vi "Gerilim_Tablo_Doldur.vi"(10 "Table Reference in":refnum<vi>, 11 "appended array in":dbl[][](array[numeric])=[[0.12345, 1.2, 0.12345], [0.12345, 1.2, 0.12345], [0.12345, 0.12345, 0.12345], [0.12345, 0.12345, 0.12345]]) -> (1 "Test Result":bool=TRUE, 2 "Table Values":string[][](array[string])=[["0,123", "0,1235"], ["0,123", "0,1235"], ["0,123", "0,1235"], ["0,123", "0,1235"], ["0,050", "0,0000"]], 3 "appended array Out":dbl[][](array[numeric])=[[0.12345, 1.2, 0.12345], [0.12345, 1.2, 0.12345], [0.12345, 0.12345, 0.12345], [0.12345, 0.12345, 0.12345], [0.049999999999999996, 0.0, 0.0]])   [LabVIEW 2014]
uses:
  TestStandInteraction/VeriPaylasim_Globali.vi
panel:
  out "OlcumNo":u16=6
  out "appended array":dbl[](array[numeric])=[0.049999999999999996, 0.0, 0.0, 0.0, 0.0, 0.0, 0.0, 0.05]
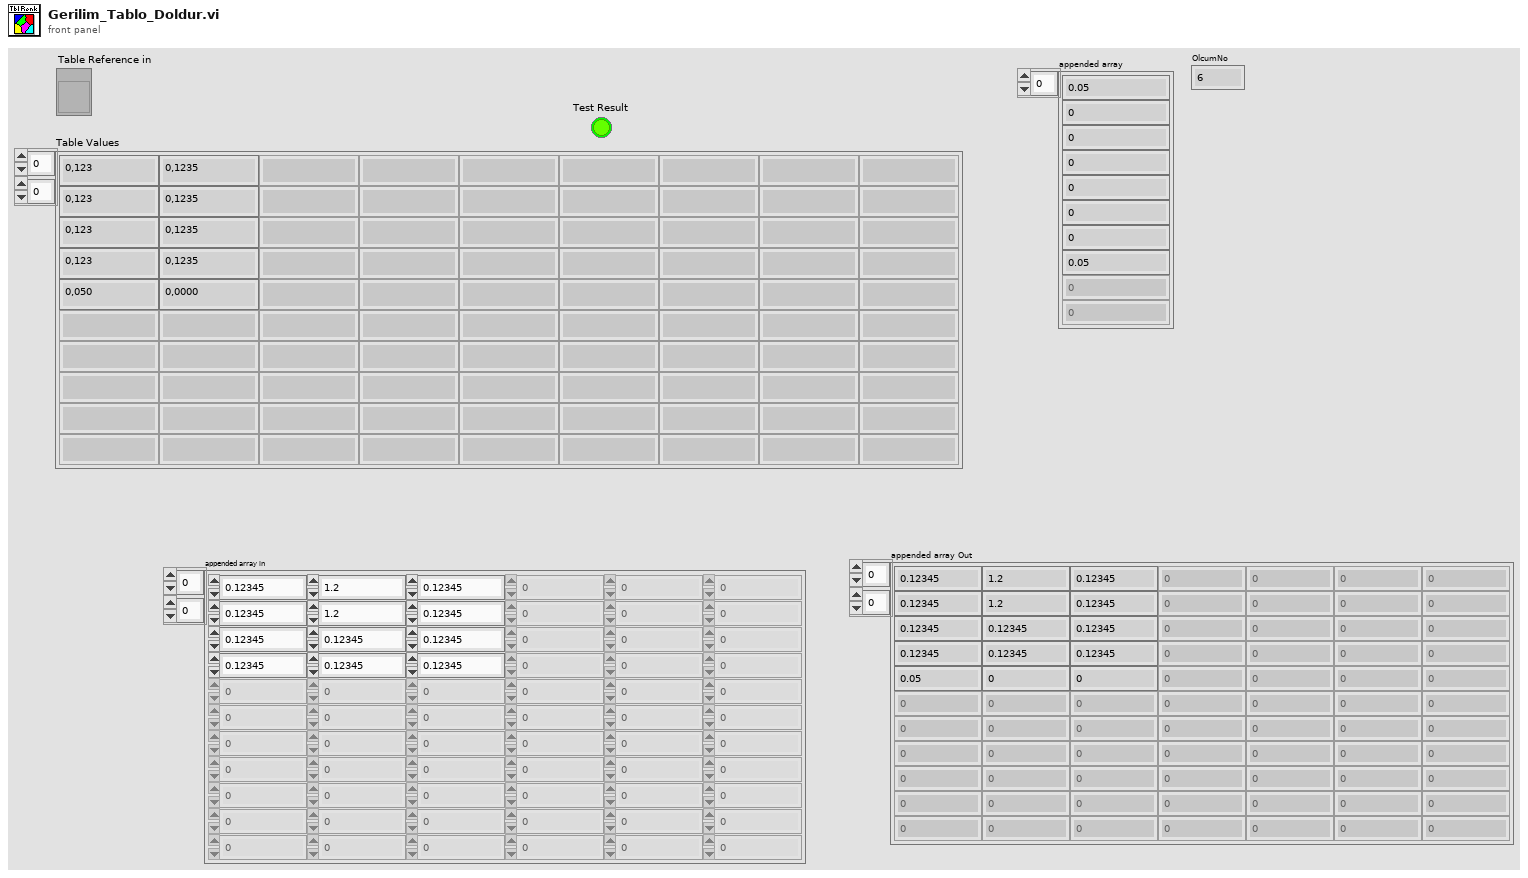
[diagram p1: front panel]
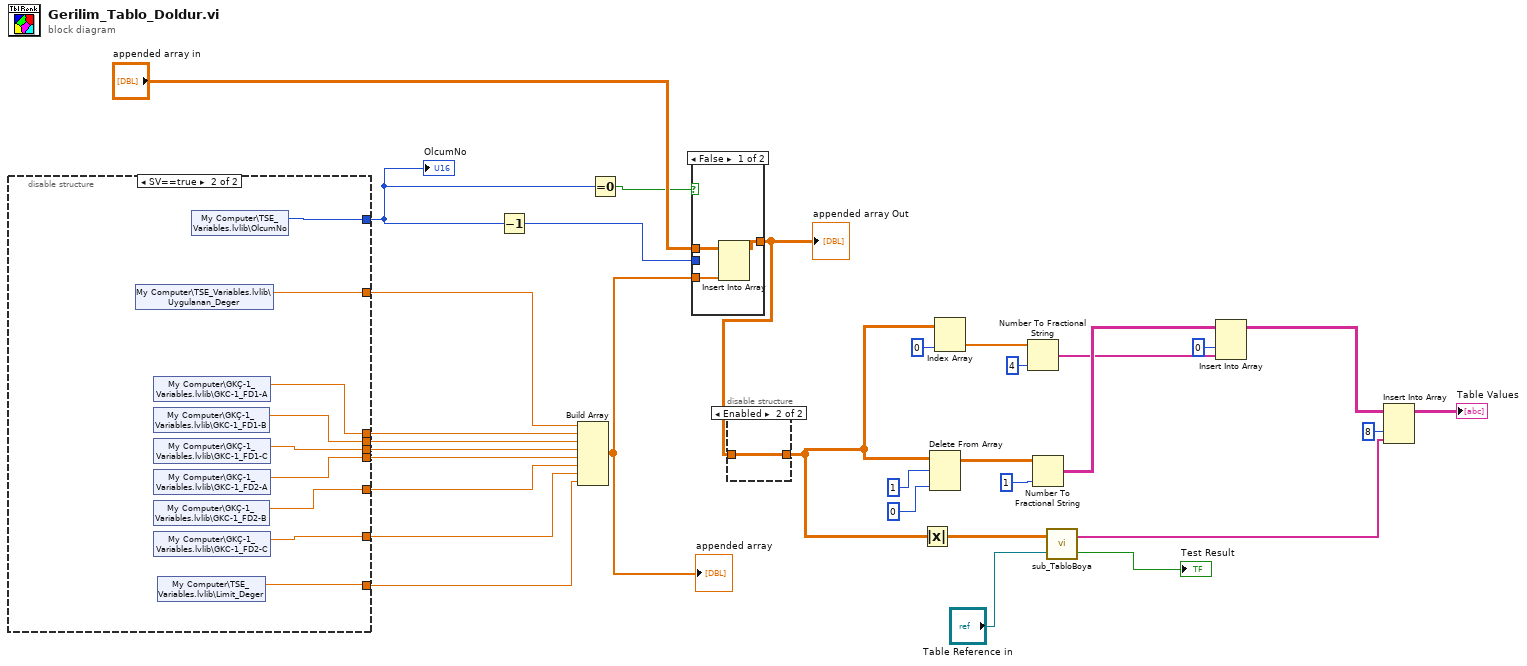
[diagram p0: block diagram]
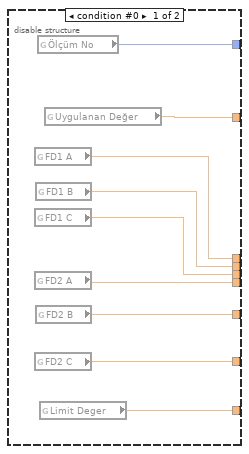
[diagram p2: hidden frame]
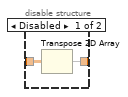
[diagram p4: hidden frame]
diagram:
  n1 = disable-structure shown="SV==true" {
    disable-tunnel: [w41 w50] -> w21
    disable-tunnel: [w40 w49] -> w20
    disable-tunnel: [w39 w47] -> w8
    disable-tunnel: [w38 w46] -> w7
    disable-tunnel: [w37 w48] -> w6
    disable-tunnel: [w36 w42] -> w5
    disable-tunnel: [w35 w43] -> w4
    disable-tunnel: [w34 w44] -> w3
    disable-tunnel: [w33 w45] -> w2
    frame condition #0 {
      n2 = global read "VeriPaylasim_Globali.vi" "FD1 A"() -> (w39:dbl)
      n3 = global read "VeriPaylasim_Globali.vi" "FD1 C"() -> (w33:dbl)
      n4 = global read "VeriPaylasim_Globali.vi" "FD2 A"() -> (w34:dbl)
      n5 = global read "VeriPaylasim_Globali.vi" "FD2 C"() -> (w36:dbl)
      n6 = global read "VeriPaylasim_Globali.vi" "FD1 B"() -> (w38:dbl)
      n7 = global read "VeriPaylasim_Globali.vi" "FD2 B"() -> (w35:dbl)
      n8 = global read "VeriPaylasim_Globali.vi" "Ölçüm No"() -> (w41:u16)
      n9 = global read "VeriPaylasim_Globali.vi" "Limit Deger"() -> (w37:dbl)
      n10 = global read "VeriPaylasim_Globali.vi" "Uygulanan Değer"() -> (w40:dbl)
    }
    frame condition #1 (active) {
      n11 = shared-variable "My Computer\\TSE_Variables.lvlib\\Uygulanan_Deger"() -> (w49:dbl)  [unwired: 1 in, 1 out]
      n12 = shared-variable "My Computer\\GKÇ-1_Variables.lvlib\\GKC-1_FD1-A"() -> (w47:dbl)  [unwired: 1 in, 1 out]
      n13 = shared-variable "My Computer\\GKÇ-1_Variables.lvlib\\GKC-1_FD1-B"() -> (w46:dbl)  [unwired: 1 in, 1 out]
      n14 = shared-variable "My Computer\\GKÇ-1_Variables.lvlib\\GKC-1_FD1-C"() -> (w45:dbl)  [unwired: 1 in, 1 out]
      n15 = shared-variable "My Computer\\GKÇ-1_Variables.lvlib\\GKC-1_FD2-A"() -> (w44:dbl)  [unwired: 1 in, 1 out]
      n16 = shared-variable "My Computer\\GKÇ-1_Variables.lvlib\\GKC-1_FD2-B"() -> (w43:dbl)  [unwired: 1 in, 1 out]
      n17 = shared-variable "My Computer\\GKÇ-1_Variables.lvlib\\GKC-1_FD2-C"() -> (w42:dbl)  [unwired: 1 in, 1 out]
      n18 = shared-variable "My Computer\\TSE_Variables.lvlib\\Limit_Deger"() -> (w48:dbl)  [unwired: 1 in, 1 out]
      n19 = shared-variable "My Computer\\TSE_Variables.lvlib\\OlcumNo"() -> (w50:u16)  [unwired: 1 in, 1 out]
    }
  }
  "OlcumNo" <- w21
  n20 = Decrement(x=w21) -> (x-1=w23:u16)
  n21 = Build Array(w20, w8, w7, w2, w3, w4, w5, w6) -> (w26:dbl[])
  "appended array" <- w26
  n22 = Equal To 0?(x=w21) -> (x = 0?=w22:bool)
  n23 = case shown="False" w22 {
    tunnel: w26 -> [w51 _]
    tunnel: [w52 w54] -> w25
    tunnel: "appended array in" -> [w53 w54]
    tunnel: w23 -> [_ _]
    frame False {
      n24 = Insert Into Array(array=w53, new element=w51) -> (w52:dbl[][])  [unwired: 2 in]
    }
    frame True {
    }
  }
  "appended array Out" <- w25
  n25 = disable-structure shown="Enabled" {
    disable-tunnel: [w56 w57] -> w17
    disable-tunnel: w25 -> [w55 w57]
    frame Disabled {
      n26 = Transpose 2D Array(2D array=w55) -> (transposed array=w56:dbl[][])
    }
    frame Enabled {
    }
  }
  n27 = Absolute Value(x=w17) -> (abs(x)=w1:dbl[][])
  n28 = Delete From Array "Delete From Array"(array=w17, length=1, index (col)=0 ("disabled index (col)")) -> (array with subset deleted=w14:dbl[][])  [unwired: 1 in, 1 out]
  n29 = Index Array "Index Array"(array=w17, index (col)=0 ("disabled index (col)")) -> (element=w18:dbl[])  [unwired: 1 in]
  n30 = Number To Fractional String(number=w18, precision (6)=i16 4) -> (F-format string=w11:string[])  [unwired: 2 in]
  n31 = Number To Fractional String(number=w14, precision (6)=i16 1) -> (F-format string=w12:string[][])  [unwired: 2 in]
  n32 = call "sub_TabloBoya.vi"("Table in"="Table Reference in", "Tablo Degerleri"=w1) -> ("Test Result"=→"Test Result":bool, "RESULTS"=w30:string[])
  n33 = Insert Into Array(array=w12, index (col)=0 ("disabled index (col)"), new element=w11) -> (w13:string[][])  [unwired: 1 in]
  n34 = Insert Into Array(array=w13, index (col)=8 ("disabled index (col)"), new element=w30) -> (→"Table Values":string[][])  [unwired: 1 in]
